vi "fullSERVER.vi"() -> ()   [LabVIEW 2023]
panel:
  in  "DAQ CHANNEL":tag
  out "SIGNAL":waveform(dbl)(graph)
  out "# POINTS":dbl
  out "OBSERVATION TIME":dbl
  out "SAMPLING FREQUENCY":dbl
  in  "PORT":u16=1500
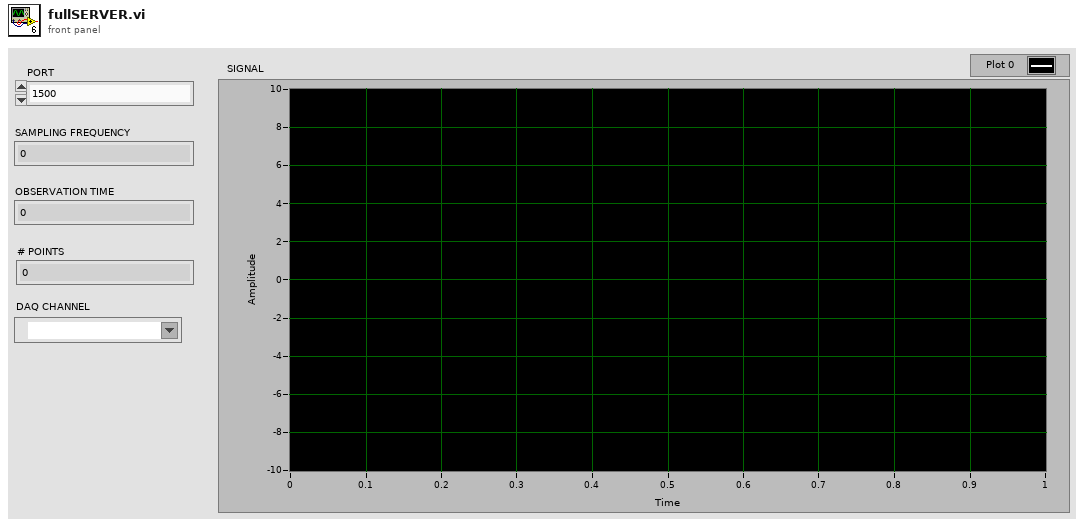
[diagram p1: front panel]
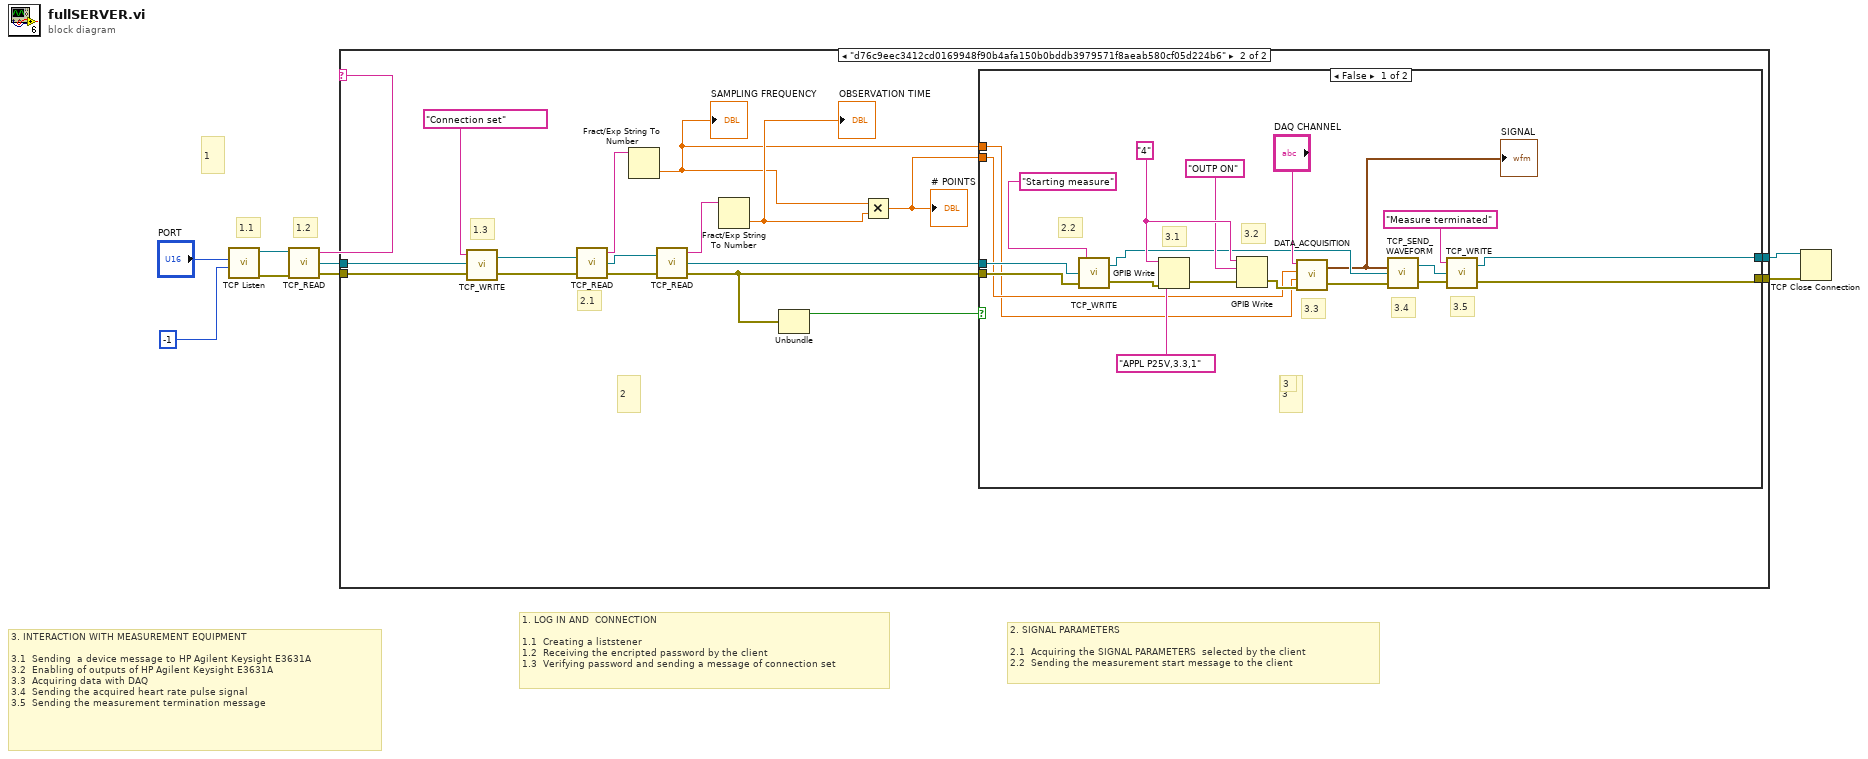
[diagram p0: block diagram]
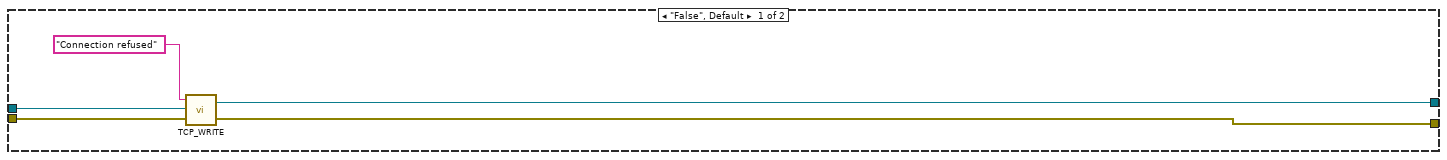
[diagram p2: hidden frame]
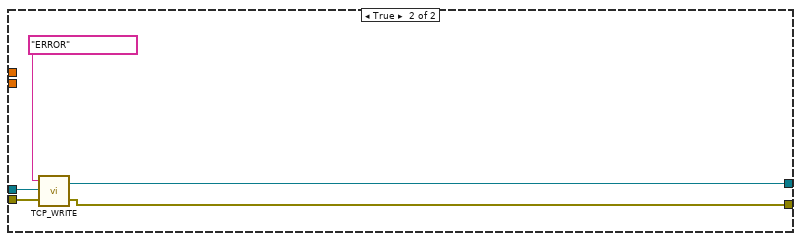
[diagram p3: hidden frame]
diagram:
  # "3. INTERACTION WITH MEASUREMENT EQUIPMENT\n\n3.1  Sending  a device message to HP Agilent Keysight E3631A       \n3.2  Enabling of outputs of HP Agilent Keysight E3631A\n3.3  Acquiring data with DAQ\n3.4  Sending the acquired heart rate pulse signal \n3.5  Sending the measurement termination message"
  # "1.2"
  # "1.1"
  # "2. SIGNAL PARAMETERS\n\n2.1  Acquiring the SIGNAL PARAMETERS  selected by the client \n2.2  Sending the measurement start message to the client"
  # "1. LOG IN AND  CONNECTION\n\n1.1  Creating a liststener\n1.2  Receiving the encripted password by the client\n1.3  Verifying password and sending a message of connection set"
  # "1"
  n1 = call <vilib>:"TCP Listen.vi"("timeout ms (wait forever: -1)"=-1, "port"="PORT") -> ("error out"=w6:errorcluster, "connection ID"=w7:refnum<k5>)  [unwired: 5 in, 3 out]
  n2 = call "TCP_READ.vi"("connection ID"=w7, "error in (no error)"=w6) -> ("data"=w5:string, "connection ID out"=w4:refnum<k5>, "error out"=w3:errorcluster)
  n3 = case shown="\"d76c9eec3412cd0169948f90b4afa150b0bddb3979571f8aeab580cf05d224b6\"" w5 {
    tunnel: w4 -> [w13 w30]
    tunnel: w3 -> [w14 w31]
    tunnel: [w12 w17] -> w2
    tunnel: [w11 w18] -> w1
    frame "False", Default {
      n4 = call "TCP_WRITE.vi"("error in (no error)"=w14, "connection ID"=w13, "data"="Connection refused") -> ("error out"=w11:errorcluster, "connection ID out"=w12:refnum<k5>)
    }
    frame "d76c9eec3412cd0169948f90b4afa150b0bddb3979571f8aeab580cf05d224b6" {
      # "2.1"
      # "1.3"
      # "2"
      n5 = call "TCP_WRITE.vi"("error in (no error)"=w31, "connection ID"=w30, "data"="Connection set") -> ("error out"=w28:errorcluster, "connection ID out"=w27:refnum<k5>)
      n6 = call "TCP_READ.vi"("connection ID"=w27, "error in (no error)"=w28) -> ("data"=w24:string, "connection ID out"=w25:refnum<k5>, "error out"=w26:errorcluster)
      n7 = Fract/Exp String To Number(string=w24) -> (number=w16:dbl)  [unwired: 3 in, 1 out]
      "SAMPLING FREQUENCY" <- w16
      n8 = call "TCP_READ.vi"("connection ID"=w25, "error in (no error)"=w26) -> ("data"=w23:string, "connection ID out"=w21:refnum<k5>, "error out"=w20:errorcluster)
      n9 = Fract/Exp String To Number(string=w23) -> (number=w22:dbl)  [unwired: 3 in, 1 out]
      "OBSERVATION TIME" <- w22
      n10 = Unbundle(w20) -> ("status"=w19:bool)  [unwired: 2 out]
      n11 = Multiply(x=w16, y=w22) -> (x*y=w15:dbl)
      "# POINTS" <- w15
      n12 = case shown="False" w19 {
        tunnel: w20 -> [w51 w56]
        tunnel: w21 -> [w50 w55]
        tunnel: [w35 w53] -> w17
        tunnel: [w34 w52] -> w18
        tunnel: w16 -> [w40 _]
        tunnel: w15 -> [w41 _]
        frame False {
          w48 = "4" ("address string")
          # "3.5"
          # "3.4"
          # "3.3"
          # "3.2"
          # "3.1"
          # "2.2"
          # "3"
          # "3"
          n13 = call "TCP_WRITE.vi"("error in (no error)"=w51, "connection ID"=w50, "data"="Starting measure") -> ("error out"=w45:errorcluster, "connection ID out"=w38:refnum<k5>)
          n14 = GPIB Write(0:w48, 1:"APPL P25V,3.3,1" ("data"), 3:w45) -> (6:w44:errorcluster)  [unwired: 2 in, 1 out]
          n15 = GPIB Write(0:w48, 1:"OUTP ON" ("data"), 3:w44) -> (6:w43:errorcluster)  [unwired: 2 in, 1 out]
          n16 = call "DATA_ACQUISITION.vi"("error in"=w43, "SAMPLING FREQ"=w40, "# SAMPLES"=w41, "DAQ CHANNEL"="DAQ CHANNEL") -> ("error out"=w39:errorcluster, "data"=w33:waveform(dbl))
          "SIGNAL" <- w33
          n17 = call "TCP_SEND_WAVEFORM.vi"("error in (no error)"=w39, "connection ID"=w38, "waveform"=w33) -> ("error out"=w37:errorcluster, "connection ID out"=w36:refnum<k5>)
          n18 = call "TCP_WRITE.vi"("error in (no error)"=w37, "connection ID"=w36, "data"="Measure terminated") -> ("error out"=w34:errorcluster, "connection ID out"=w35:refnum<k5>)
        }
        frame True {
          n19 = call "TCP_WRITE.vi"("error in (no error)"=w56, "connection ID"=w55, "data"="ERROR") -> ("error out"=w52:errorcluster, "connection ID out"=w53:refnum<k5>)
        }
      }
    }
  }
  n20 = TCP Close Connection(connection ID=w2, error in (no error)=w1) -> ()  [unwired: 1 in, 2 out]
